vi "Relink Test.vi"() -> ()   [LabVIEW 2017]
uses:
  <vilib>/gpm_packages/@cs/test-executive/Source/Test Executive/TestExecutive/Test Executive.lvclass
  C:/Program Files/National Instruments/LabVIEW 2017/vi.lib/gpm_packages/@cs/test-executive/Source/Test Executive/ITestExecutive/ITest Executive.lvclass
  <vilib>/gpm_packages/@cs/test-executive/Source/Path Builder/IPath Builder/IPath Builder.lvclass
  <vilib>/gpm_packages/@cs/test-executive/Source/Compatibility Helper/ICompatibility Helper.lvclass
  <vilib>/gpm_packages/@cs/persistence/source/XML/XML.lvclass
  C:/Program Files/National Instruments/LabVIEW 2017/vi.lib/gpm_packages/@cs/persistence/source/IPersist/IPersist.lvclass
  <vilib>/gpm_packages/@cs/test-executive/Source/Test Executive/TestExecutive Ref/TestExecutive Ref.lvclass
panel:
  out "error out":errorcluster
  in  "Tree":string(tree)
  out "Return":string
  in  "File":path
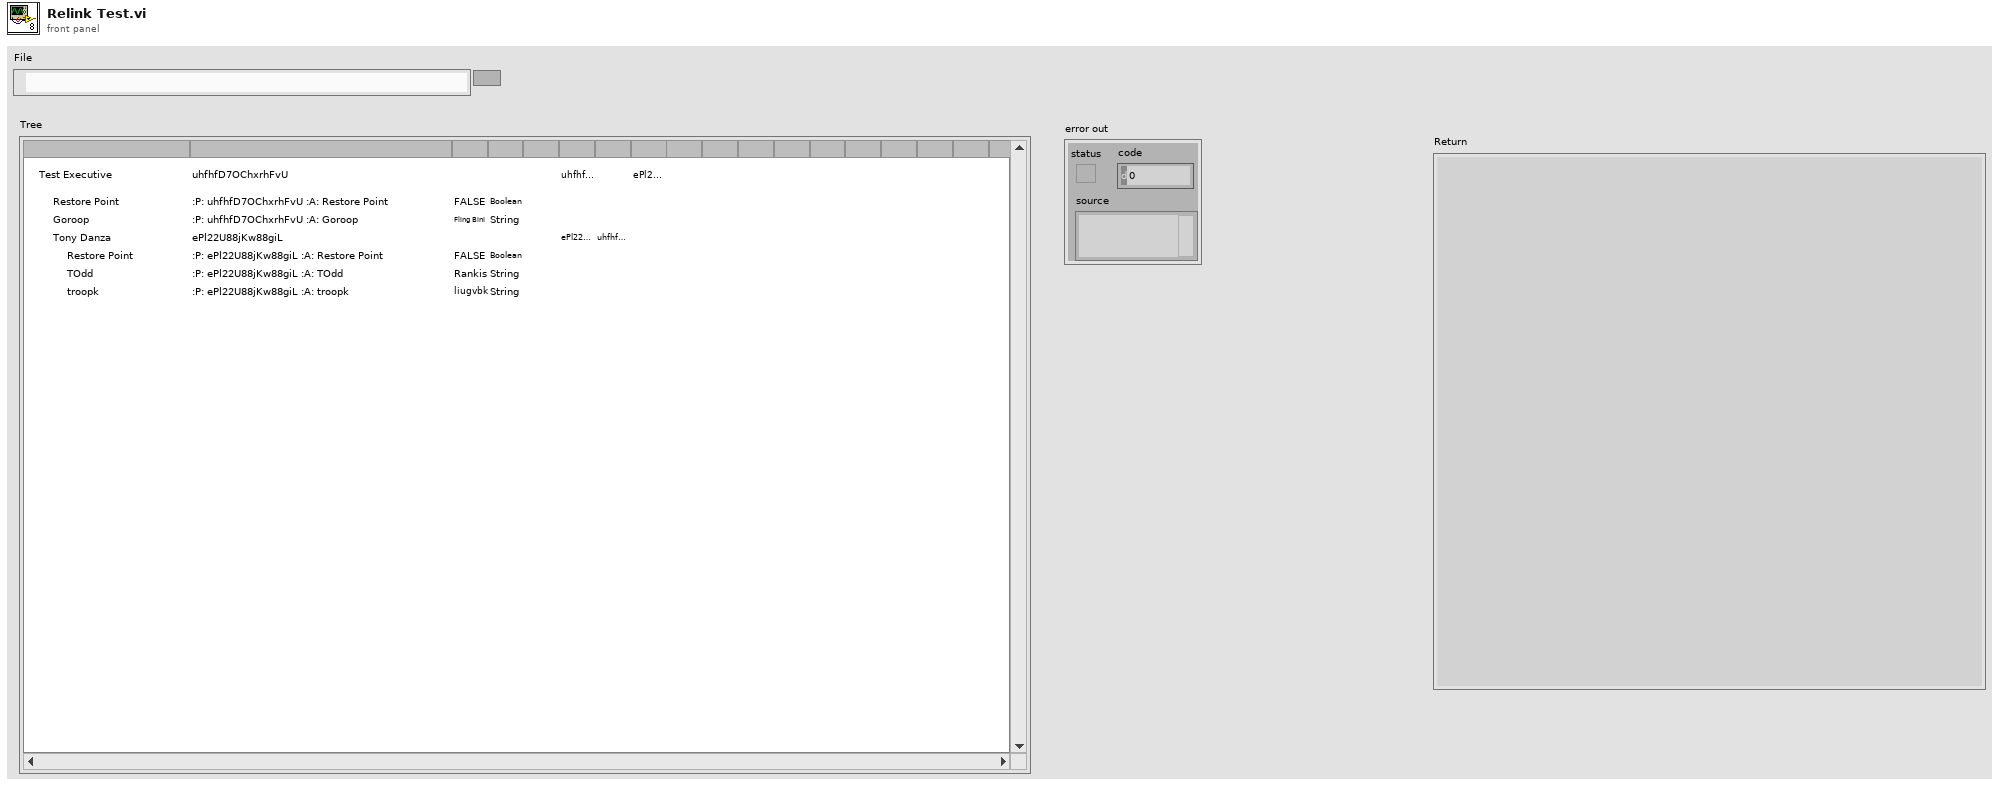
[diagram p1: front panel]
types:
  T1 = cluster{"Left Cell String":string, "Child Text":string[], "Child Tag":string, "Item Indent":i32, "Child Only?":bool, "Glyph Index":i32}[]
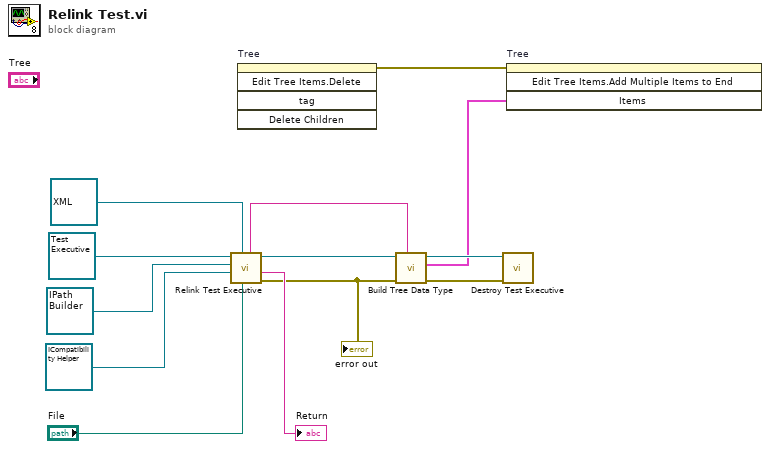
[diagram p0: block diagram]
diagram:
  n1 = call <vilib>:"Relink Test Executive.vi"("File"="File", "Persistence in"=refnum<class "XML.lvclass"> refnum ("XML.lvlib:XML.lvclass"), "Compatibility Helper"=refnum<class "ICompatibility Helper.lvclass"> refnum, "Path Builder"=refnum<class "IPath Builder.lvclass"> refnum, "Test Executive"=refnum<class "Test Executive.lvclass"> refnum ("Test Executive.lvlib:Test Executive.lvclass")) -> ("error out"=w6:errorcluster, "Return"=→"Return":string, "Test Executive Ref out"=w7:refnum<data-value>, "Root ID"=w1:string)  [unwired: 3 in]
  "error out" <- w6
  n2 = invoke on="Tree" class="Tree (strict)" method="Edit Tree Items.Delete"() -> (error out=w3:errorcluster)  [unwired: 5 in, 4 out]
  n3 = call <vilib>:"Build Tree Data Type.vi"("Test ID"=w1, "error in (no error)"=w6, "Test Executive Ref"=w7) -> ("error out"=w4:errorcluster, "Tree Data"=w2:T1, "Test Executive Ref out"=w5:refnum<data-value>)  [unwired: 6 in]
  n4 = call <vilib>:"Destroy Test Executive.vi"("error in (no error)"=w4, "Test Executive Ref"=w5) -> ()  [unwired: 9 in, 1 out]
  n5 = invoke on="Tree" class="Tree (strict)" method="Edit Tree Items.Add Multiple Items to End"(error in=w3, "Items"=w2) -> ()  [unwired: 2 in, 4 out]
